vi "FPGA_DIOReadFilterPeriod.vi"(6 "DIOChannel":T1, 8 "error in (no error)":errorcluster, 10 "index":u8, 11 "DIODeviceRef In":T2) -> (0 "error out":errorcluster, 2 "PWMFilterPeriod":u32, 3 "DIODeviceRef Out":T2)   [LabVIEW 2017]
uses:
  <vilib>/Rock Robotics/SystemInterfaces/DIO/FPGA_DIODevRef.ctl
  <vilib>/Rock Robotics/SystemInterfaces/DIO/FPGA_DIOChannel.ctl
  <vilib>/Rock Robotics/SystemInterfaces/System/FPGA_SystemFPGA Ref Global.vi
  <vilib>/Utility/error.llb/Error Cluster From Error Code.vi
  <vilib>/rvi/errors/niLvFpgaAdjustHostInterfaceError.vi
  <vilib>/rvi/interface/nirviReadWriteControl/nirviReadWriteControl.xnode
  <vilib>/Rock Robotics/SystemInterfaces/System/FPGA_SystemFRC FPGA Ref.ctl
  NiFpgaLv.dll
  <vilib>/rvi/interface/Simulation/niFpgaSimulationCallBeginRW.vi
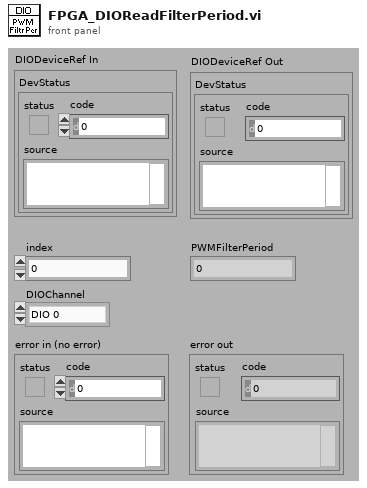
[diagram p1: front panel]
types:
  T1 = typedef "FPGA_DIOChannel.ctl" = enum8{"DIO 0", "DIO 1", "DIO 2", "DIO 3", "DIO 4", "DIO 5", "DIO 6", "DIO 7", "DIO 8", "DIO 9", "DIO MXP 0", "DIO MXP 1", "DIO MXP 2", "DIO MXP 3", "DIO MXP 4", "DIO MXP 5", "DIO MXP 6", "DIO MXP 7", "DIO MXP 8", "DIO MXP 9", "DIO MXP 10", "DIO MXP 11", "DIO MXP 12", "DIO MXP 13", "DIO MXP 14", "DIO MXP 15", "SPI Port CS1", "SPI Port CS2", "SPI Port CS3", "SPI Port MISO", "SPI Port MOSI", "Invalid"}
  T2 = typedef "FPGA_DIODevRef.ctl" = cluster{"DevStatus":errorcluster}
  T3 = typedef "FPGA_SystemFRC FPGA Ref.ctl" = refnum<k20>
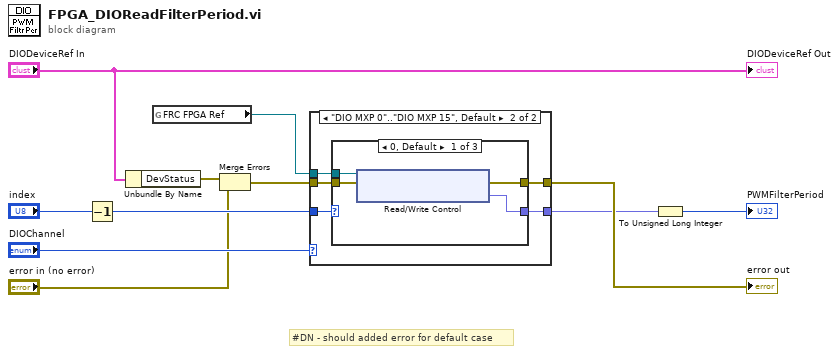
[diagram p0: block diagram]
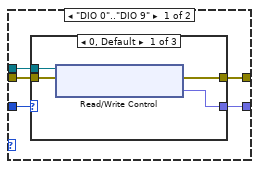
[diagram p2: hidden frame]
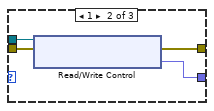
[diagram p3: hidden frame]
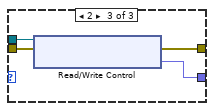
[diagram p4: hidden frame]
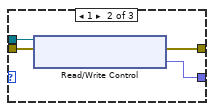
[diagram p5: hidden frame]
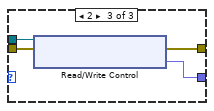
[diagram p6: hidden frame]
diagram:
  # "#DN - should added error for default case"
  n1 = Decrement(x="index") -> (x-1=w4:u8)
  n2 = Unbundle By Name("DIODeviceRef In") -> ("DevStatus"=w7:errorcluster)
  n3 = global read "FPGA_SystemFPGA Ref Global.vi" "FRC FPGA Ref"() -> (w8:T3)
  n4 = Merge Errors(w7, "error in (no error)") -> (w6:errorcluster)
  n5 = case shown="\"DIO MXP 0\"..\"DIO MXP 15\", Default" "DIOChannel" {
    tunnel: [w16 w33] -> w11
    tunnel: [w13 w30] -> w9
    tunnel: w8 -> [w15 w32]
    tunnel: w6 -> [w14 w31]
    tunnel: w4 -> [w12 w29]
    frame "DIO 0".."DIO 9" {
      n6 = case shown="0, Default" w12 {
        tunnel: [w20 w24 w28] -> w16
        tunnel: w15 -> [w19 w23 w27]
        tunnel: w14 -> [w18 w22 w26]
        tunnel: [w17 w21 w25] -> w13
        frame 0, Default {
          n7 = xnode "Read/Write Control"("FPGA VI Reference In"=w19, "error in"=w18) -> ("error out"=w20:errorcluster, "DIO.FilterPeriodHdr0"=w17:fxp<+,24,24>)  [unwired: 1 out]
        }
        frame 1 {
          n8 = xnode "Read/Write Control"("FPGA VI Reference In"=w23, "error in"=w22) -> ("error out"=w24:errorcluster, "DIO.FilterPeriodHdr1"=w21:fxp<+,24,24>)  [unwired: 1 out]
        }
        frame 2 {
          n9 = xnode "Read/Write Control"("FPGA VI Reference In"=w27, "error in"=w26) -> ("error out"=w28:errorcluster, "DIO.FilterPeriodHdr2"=w25:fxp<+,24,24>)  [unwired: 1 out]
        }
      }
    }
    frame "DIO MXP 0".."DIO MXP 15", Default {
      n10 = case shown="0, Default" w29 {
        tunnel: [w37 w41 w45] -> w33
        tunnel: w32 -> [w36 w40 w44]
        tunnel: w31 -> [w35 w39 w43]
        tunnel: [w34 w38 w42] -> w30
        frame 0, Default {
          n11 = xnode "Read/Write Control"("FPGA VI Reference In"=w36, "error in"=w35) -> ("error out"=w37:errorcluster, "DIO.FilterPeriodMXP0"=w34:fxp<+,24,24>)  [unwired: 1 out]
        }
        frame 1 {
          n12 = xnode "Read/Write Control"("FPGA VI Reference In"=w40, "error in"=w39) -> ("error out"=w41:errorcluster, "DIO.FilterPeriodMXP1"=w38:fxp<+,24,24>)  [unwired: 1 out]
        }
        frame 2 {
          n13 = xnode "Read/Write Control"("FPGA VI Reference In"=w44, "error in"=w43) -> ("error out"=w45:errorcluster, "DIO.FilterPeriodMXP2"=w42:fxp<+,24,24>)  [unwired: 1 out]
        }
      }
    }
  }
  "error out" <- w11
  n14 = To Unsigned Long Integer(number=w9) -> (unsigned 32bit integer=→"PWMFilterPeriod":u32)
  "DIODeviceRef Out" <- "DIODeviceRef In"
